vi "TcA06-004_ObjectsAreDestroyedEvenIfErrorIn.vi"(1 "Input buffer":T3="1", 3 "Invocation info":T2, 5 "error in (no error)":errorcluster, 6 "Add log to result?":bool) -> (16 "Test Data":T1 {"Numeric Measurement" format="%.2f"}, 19 "error out":errorcluster)   [LabVIEW 2009]
doc: "Test case template."
uses:
  Shared/Support_InputBuffer.ctl
  Shared/Support_InvocationInfo.ctl
  Shared/Support_TestData.ctl
  TestClasses/G#BaseClass2_class/G#BaseClass2.lvclass
  TestClasses/G#SubSubClass2_class/G#SubSubClass2.lvclass
  TestClasses/G#BaseClass1_class/G#BaseClass1.lvclass
  <vilib>/addons/_AddQ/G#Object/G#Object.lvclass
panel:
  in  "Test name":string="TcA06-004 Objects are destroyed even if error in"
  out "Test result":bool
  out "Result":string
  # "Verify that objects are destroyed even if there is an error in\nto the destructor."
  # "Sub test case"
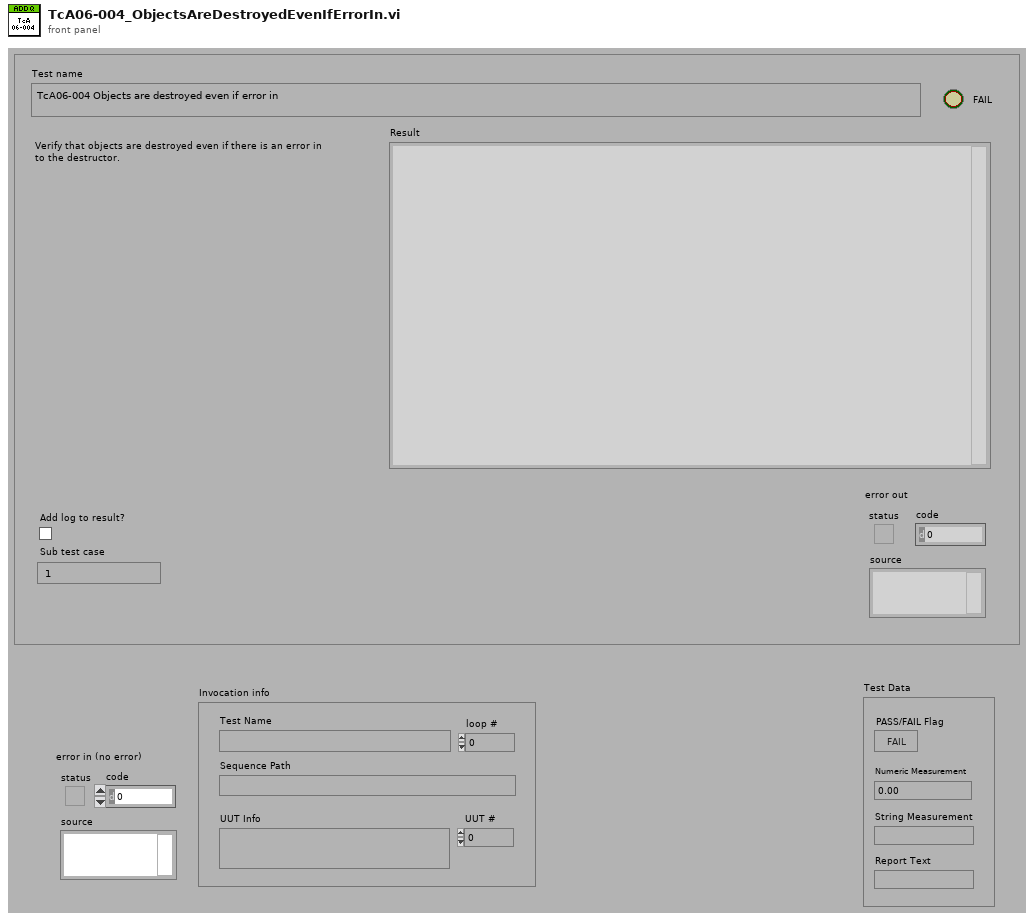
[diagram p1: front panel]
types:
  T1 = typedef "Support_TestData.ctl" = cluster{"PASS/FAIL Flag":bool, "Numeric Measurement":dbl, "String Measurement":string, "Report Text":string}
  T2 = typedef "Support_InvocationInfo.ctl" = cluster{"UUT #":i32, "loop #":i32, "UUT Info":string, "Test Name":string, "Sequence Path":path}
  T3 = typedef "Support_InputBuffer.ctl" = string
  T4 = typedef "Support_ResultType.ctl" = cluster{"Pass":bool, "Comment":string, "MeasurementValue":dbl}
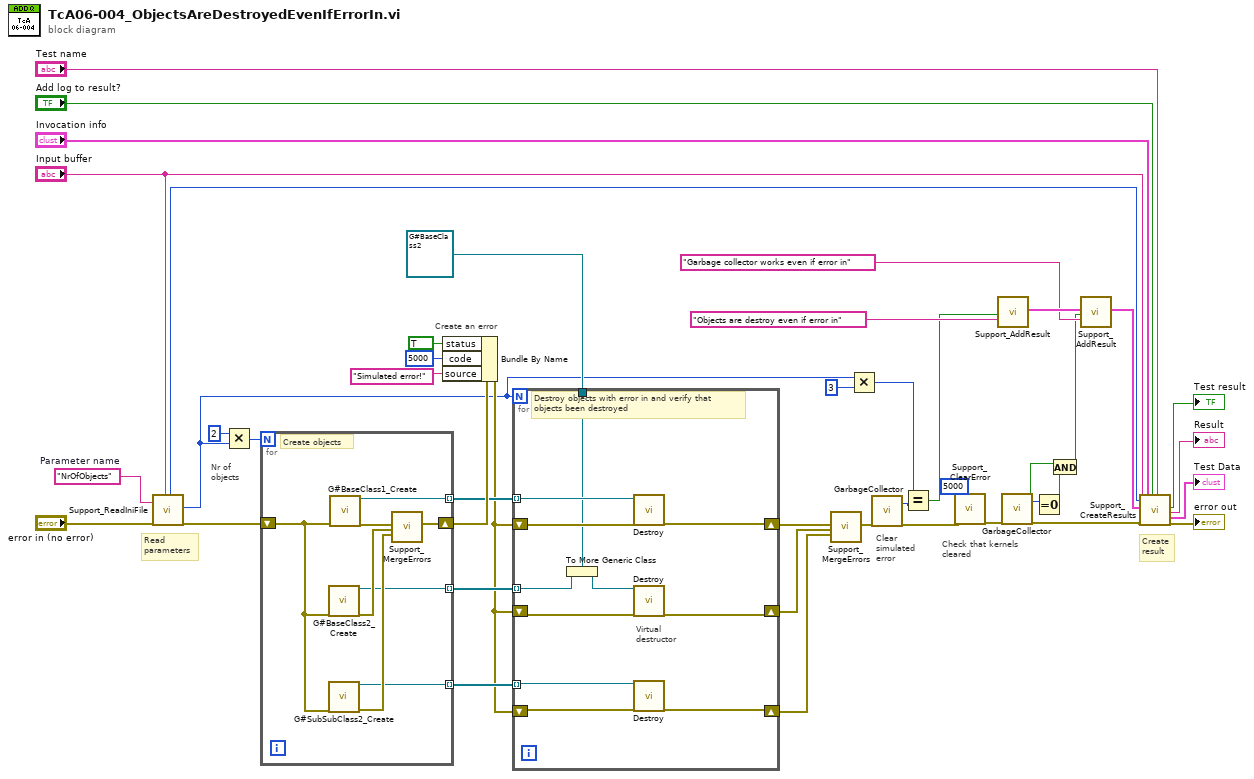
[diagram p0: block diagram]
diagram:
  w38 = "NrOfObjects"  # Parameter name
  # "Clear\nsimulated\nerror"
  # "Check that kernels\ncleared"
  # "Create an error"
  # "Nr of\nobjects"
  # "Create\nresult"
  # "Read\nparameters"
  n1 = call "Support_ReadIniFile.vi"("Parameter name"=w38, "error in (no error)"="error in (no error)", "Sub test case"="Input buffer") -> ("Timer start"=w34:u32, "Parameter1 as I32"=w1:i32, "error out"=w33:errorcluster)  [unwired: 9 in, 5 out]
  n2 = Multiply(x=2, y=w1) -> (x*y=w14:i32)
  n3 = for {
    N: w14 -> [_]
    shift-right: [w50] -> w27
    shift-left: w33 -> [w52]
    tunnel: [w47] -> w29 mode=indexing
    tunnel: [w46] -> w28 mode=indexing
    tunnel: [w45] -> w26 mode=indexing
    # "Create objects"
    n4 = call "G#BaseClass2_Create.vi"("error in (no error)"=w52) -> ("reference out"=w47:refnum<class "G#BaseClass2.lvclass">, "error out"=w49:errorcluster)  [unwired: 17 in]
    n5 = call "G#SubSubClass2_Create.vi"("error in (no error)"=w52) -> ("reference out"=w46:refnum<class "G#SubSubClass2.lvclass">, "error out"=w48:errorcluster)  [unwired: 17 in]
    n6 = call "G#BaseClass1_Create.vi"("error in (no error)"=w52) -> ("reference out"=w45:refnum<class "G#BaseClass1.lvclass">, "error out"=w51:errorcluster)  [unwired: 16 in, 1 out]
    n7 = call "Support_MergeErrors.vi"("error in 1"=w51, "error in 2"=w49, "error in 3"=w48) -> ("error out"=w50:errorcluster)  [unwired: 15 in, 1 out]
  }
  n8 = Bundle By Name(cluster=w27, "status"=TRUE, "code"=5000, "source"="Simulated error!") -> (w20:errorcluster)
  n9 = for {
    N: w1 -> [_]
    shift-right: [w60] -> w23
    shift-left: w20 -> [w61]
    tunnel: w29 -> [w55] mode=indexing
    tunnel: w28 -> [w63] mode=indexing
    tunnel: w26 -> [w62] mode=indexing
    shift-right: [w59] -> w22
    shift-left: w20 -> [w56]
    shift-right: [w58] -> w21
    shift-left: w20 -> [w57]
    tunnel: refnum<class "G#BaseClass2.lvclass"> refnum ("G#BaseClass2.lvclass") -> [w53]
    # "Virtual\ndestructor"
    # "Destroy objects with error in and verify that\nobjects been destroyed"
    n10 = To More Generic Class(target class=w53, reference=w55) -> (generic class reference=w54:refnum<class "G#BaseClass2.lvclass">)
    n11 = call-dynamic "Destroy.vi"("reference in"=w62, "error in (no error)"=w61) -> ("error out"=w60:errorcluster)  [unwired: 16 in, 1 out]
    n12 = call-dynamic "Destroy.vi"("reference in"=w54, "error in (no error)"=w56) -> ("error out"=w59:errorcluster)  [unwired: 16 in, 1 out]
    n13 = call-dynamic "Destroy.vi"("reference in"=w63, "error in (no error)"=w57) -> ("error out"=w58:errorcluster)  [unwired: 16 in, 1 out]
  }
  n14 = call "Support_MergeErrors.vi"("error in 1"=w23, "error in 2"=w22, "error in 3"=w21) -> ("error out"=w17:errorcluster)  [unwired: 15 in, 1 out]
  n15 = Multiply(x=w1, y=3) -> (x*y=w3:i32)
  n16 = call <vilib>:"GarbageCollector.vi"("error in (no error)"=w17) -> ("# of objects killed"=w12:i32, "error out"=w18:errorcluster)  [unwired: 16 in, 1 out]
  n17 = Equal?(x=w3, y=w12) -> (x = y?=w10:bool)
  n18 = call "Support_ClearError.vi"("code"=5000, "error in (no error)"=w18) -> ("error out"=w9:errorcluster)  [unwired: 16 in, 1 out]
  n19 = call "Support_AddResult.vi"("Pass"=w10, "Comment"="Objects are destroy even if error in") -> ("Results out"=w16:T4[])  [unwired: 17 in]
  n20 = call <vilib>:"GarbageCollector.vi"("error in (no error)"=w9) -> ("OK"=w6:bool, "# of objects killed"=w7:i32, "error out"=w8:errorcluster)  [unwired: 16 in]
  n21 = Equal To 0?(x=w7) -> (x = 0?=w5:bool)
  n22 = And(x=w6, y=w5) -> (x .and. y?=w4:bool)
  n23 = call "Support_AddResult.vi"("Results in"=w16, "Pass"=w4, "Comment"="Garbage collector works even if error in") -> ("Results out"=w15:T4[])  [unwired: 16 in]
  n24 = call "Support_CreateResults.vi"("Sub test case"="Input buffer", "Timer start"=w34, "Results"=w15, "error in (no error)"=w8, "Invocation info"="Invocation info", "Add log to result?"="Add log to result?", "Test name"="Test name") -> ("Pass/fail flag"=→"Test result":bool, "Result"=→"Result":string, "Test Data"=→"Test Data":T1, "error out"=→"error out":errorcluster)  [unwired: 9 in]
